vi "Find roboRIO.vi"(8 "error in (no error)":errorcluster, 10 "Queue In":refnum<queue>, 11 "UI Data in":T1) -> (0 "error out":errorcluster, 3 "UI Data out":T1)   [LabVIEW 2018, in "Personalities Tool.lvlib"]
doc: "This subVI looks for a roboRIO and selects the loaded personality for it."
uses:
  Personalities Tool.lvlib
  Controls/QMH Data.ctl
  Controls/Personality Type.ctl
  Controls/roboRIO Connection Information.ctl
  Message Queue/Message Cluster.ctl
  Message Queue/Enqueue Message (Single).vi
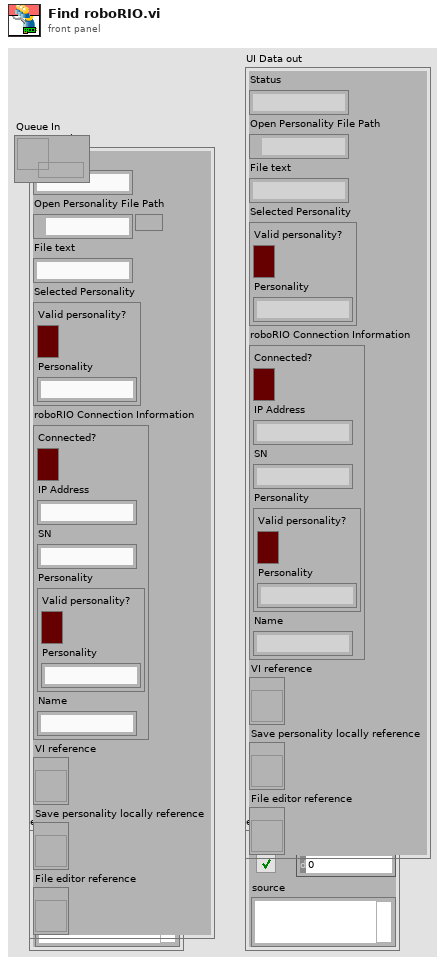
[diagram p1: front panel]
types:
  T1 = typedef "Personalities Tool.lvlib/QMH Data.ctl" = cluster{"Status":string, "Open Personality File Path":path, "File text":string, "Selected Personality":T2, "roboRIO Connection Information":T3, "VI reference":refnum<vi>, "Save personality locally reference":refnum<vi>, "File editor reference":refnum<vi>}
  T2 = typedef "Personalities Tool.lvlib/Personality Type.ctl" = cluster{"Valid personality?":bool, "Personality":string}
  T3 = typedef "Personalities Tool.lvlib/roboRIO Connection Information.ctl" = cluster{"Connected?":bool, "IP Address":string, "SN":string, "Personality":T2, "Name":string}
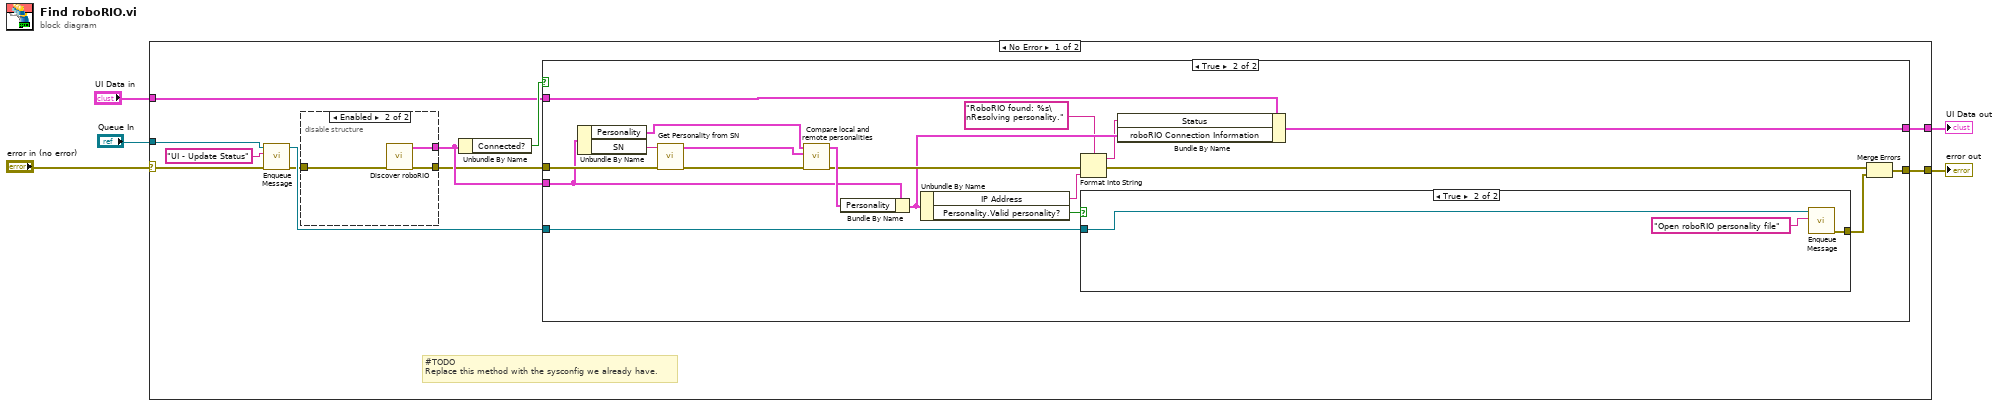
[diagram p0: block diagram]
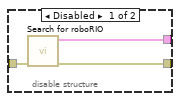
[diagram p2: hidden frame]
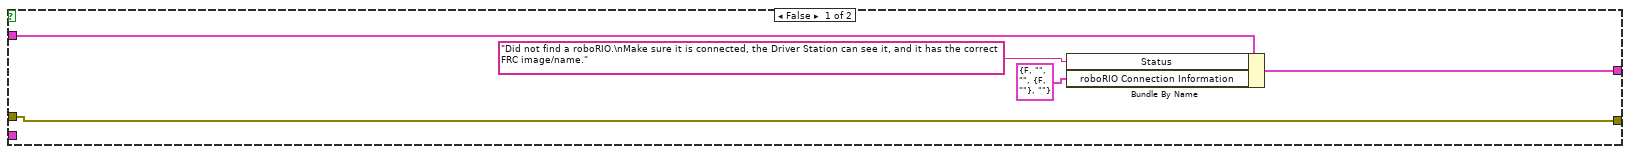
[diagram p3: hidden frame]
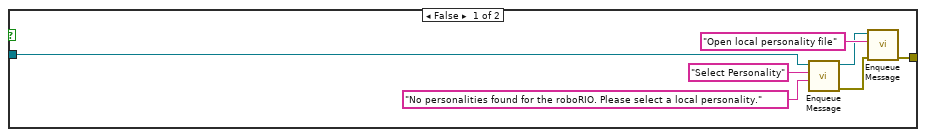
[diagram p4: hidden frame]
diagram:
  n1 = case shown="No Error" "error in (no error)" {
    selector: "error in (no error)" -> [w12 w58]
    tunnel: [w10 w58] -> w4
    tunnel: [w8 w57] -> w3
    tunnel: "UI Data in" -> [w7 w57]
    tunnel: "Queue In" -> [w6 _]
    frame No Error {
      # "#TODO\nReplace this method with the sysconfig we already have."
      n2 = call-poly "Enqueue Message.vi"("error in (no error)"=w12, "Message"="UI - Update Status", "Message Queue"=w6) -> ("error out"=w13:errorcluster, "dup Message Queue"=w14:refnum<queue>)  [unwired: 7 in]
      n3 = disable-structure shown="Enabled" {
        disable-tunnel: [w19 w20] -> w15
        disable-tunnel: w13 -> [w18 w22]
        disable-tunnel: [w17 w21] -> w9
        frame Disabled {
          n4 = call "Search for roboRIO.vi"("error in (no error)"=w18) -> ("error out"=w17:errorcluster, "roboRIO Connection Information"=w19:T3)  [unwired: 9 in]
        }
        frame Enabled {
          n5 = call "Discover roboRIO.vi"("error in (no error)"=w22) -> ("error out"=w21:errorcluster, "roboRIO Connection Information out"=w20:T3)  [unwired: 9 in]
        }
      }
      n6 = Unbundle By Name(w15) -> ("Connected?"=w16:bool)
      n7 = case shown="True" w16 {
        tunnel: w7 -> [w27 w46]
        tunnel: [w26 w45] -> w8
        tunnel: w9 -> [w23 w44]
        tunnel: [w23 w35] -> w10
        tunnel: w14 -> [_ w33]
        tunnel: w15 -> [_ w32]
        frame False {
          n8 = Bundle By Name(cluster=w27, "Status"="Did not find a roboRIO.\nMake sure it is connected, the Driver Station can see it, and it has the correct FRC image/name.", "roboRIO Connection Information"=T3 {"Connected?"=FALSE, "IP Address"="", "SN"="", "Personality"={"Valid personality?"=FALSE, "Personality"=""}, "Name"=""}) -> (w26:T1)
        }
        frame True {
          n9 = Unbundle By Name(w32) -> ("Personality"=w42:T2, "SN"=w43:string)
          n10 = call "Get Personality from SN.vi"("error in (no error)"=w44, "SN"=w43) -> ("error out"=w39:errorcluster, "DB personality"=w41:T2)  [unwired: 8 in]
          n11 = call "Compare local and remote personalities.vi"("error in (no error)"=w39, "DB personality"=w41, "roboRIO personality"=w42) -> ("error out"=w38:errorcluster, "Loaded Personality"=w40:T2)  [unwired: 7 in]
          n12 = Bundle By Name(cluster=w32, "Personality"=w40) -> (w37:T3)
          n13 = Unbundle By Name(w37) -> ("IP Address"=w28:string, "Personality.Valid personality?"=w36:bool)
          n14 = Format Into String(format string="RoboRIO found: %s\nResolving personality." ("Status"), error in=w38, w28) -> (resulting string=w30:string, error out=w31:errorcluster)  [unwired: 1 in]
          n15 = case shown="True" w36 {
            tunnel: w33 -> [w53 w55]
            tunnel: [w47 w54] -> w34
            frame False {
              n16 = call-poly "Enqueue Message.vi"("Message Data"="No personalities found for the roboRIO. Please select a local personality." ("UI message"), "Message"="Select Personality", "Message Queue"=w53) -> ("error out"=w48:errorcluster, "dup Message Queue"=w49:refnum<queue>)  [unwired: 7 in]
              n17 = call-poly "Enqueue Message.vi"("error in (no error)"=w48, "Message"="Open local personality file", "Message Queue"=w49) -> ("error out"=w47:errorcluster)  [unwired: 7 in, 1 out]
            }
            frame True {
              n18 = call-poly "Enqueue Message.vi"("Message"="Open roboRIO personality file", "Message Queue"=w55) -> ("error out"=w54:errorcluster)  [unwired: 8 in, 1 out]
            }
          }
          n19 = Bundle By Name(cluster=w46, "Status"=w30, "roboRIO Connection Information"=w37) -> (w45:T1)
          n20 = Merge Errors(w31, w34) -> (w35:errorcluster)
        }
      }
    }
    frame Error {
    }
  }
  "error out" <- w4
  "UI Data out" <- w3
